vi "setBoardNumber.vi"(8 "error in (no error)":errorcluster, 10 "boardNumber":i32, 11 "SpinCore in":refnum<class "SpinCore.lvclass">) -> (0 "error out":errorcluster, 3 "SpinCore out":refnum<class "SpinCore.lvclass">)   [LabVIEW 2011, in "Hardware.lvlib" / "Channels.lvlib" / "SpinCore.lvclass"]
uses:
  SpinCore.lvclass
  SpinCore.lvclass/SpinCore.ctl
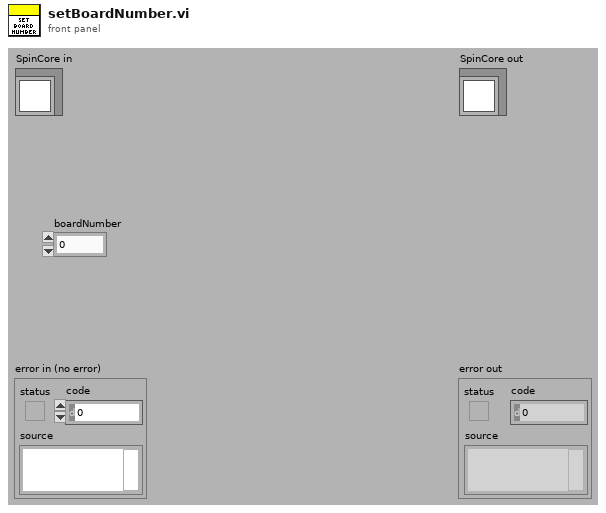
[diagram p1: front panel]
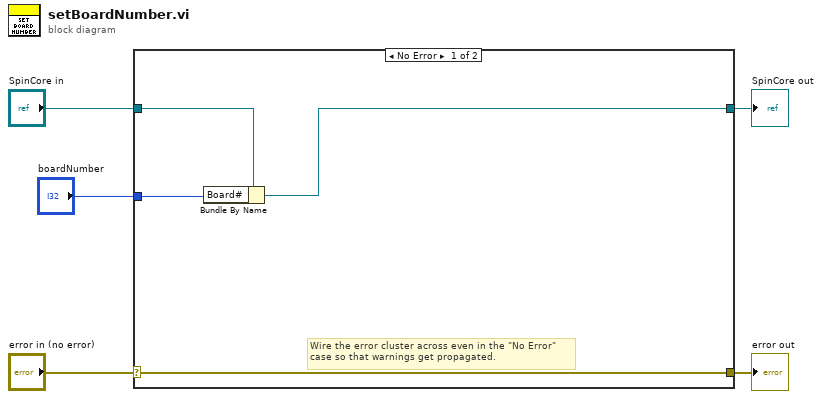
[diagram p0: block diagram]
diagram:
  n1 = case shown="No Error" "error in (no error)" {
    selector: "error in (no error)" -> [w9 w11]
    tunnel: [w9 w11] -> w4
    tunnel: [w6 w10] -> w2
    tunnel: "SpinCore in" -> [w7 w10]
    tunnel: "boardNumber" -> [w8 _]
    frame No Error {
      # "Wire the error cluster across even in the \"No Error\"\ncase so that warnings get propagated."
      n2 = Bundle By Name(cluster=w7, "Board#"=w8) -> (w6:refnum<class "SpinCore.lvclass">)
    }
    frame Error {
    }
  }
  "error out" <- w4
  "SpinCore out" <- w2
